vi "GV z stage as trigger.vi"() -> ()   [LabVIEW 2017]
panel:
  out "ZstageAsTrig":bool
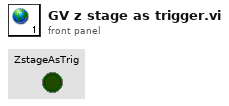
[diagram p1: front panel]
diagram:
